vi "NET_1 (1).vi"() -> ()   [LabVIEW 2017]
uses:
  <vilib>/ErrorRing/Error Ring.xnode
panel:
  out "Gauge":dbl(knob) scale=0.0..10.0
  out "Array 2":dbl[](array[numeric])
  out "output array 2":dbl[][](array[numeric])
  out "Array":u32[](array[numeric])
  out "Numeric":u32
  out "subarray":string[](array[string])
  out "Trama":string[](array[string])
  in  "Al 3":bool
  in  "Al 2":bool
  in  "Al1":bool
  in  "Escribir":bool
  out "IsOpen":bool
  in  "stop":bool
  in  "Cerrar":bool
  in  "Abrir":bool
  in  "Puertos":string(combo)
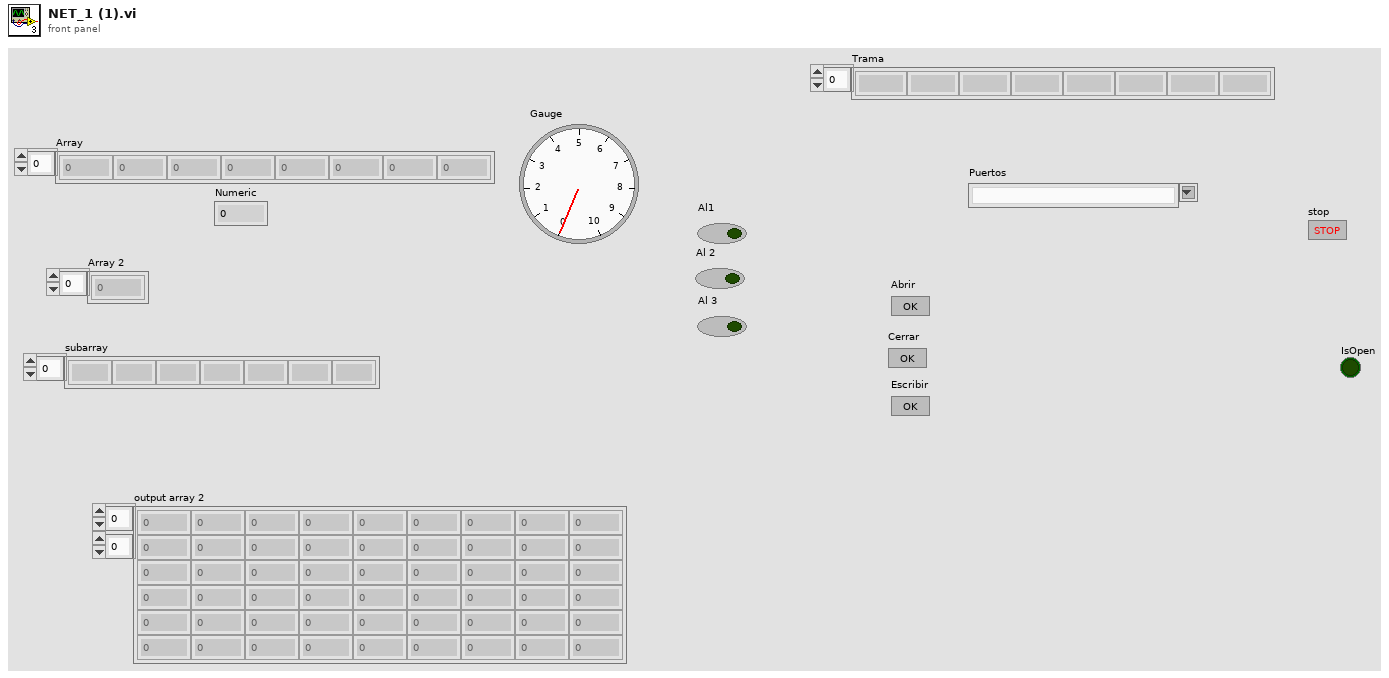
[diagram p1: front panel]
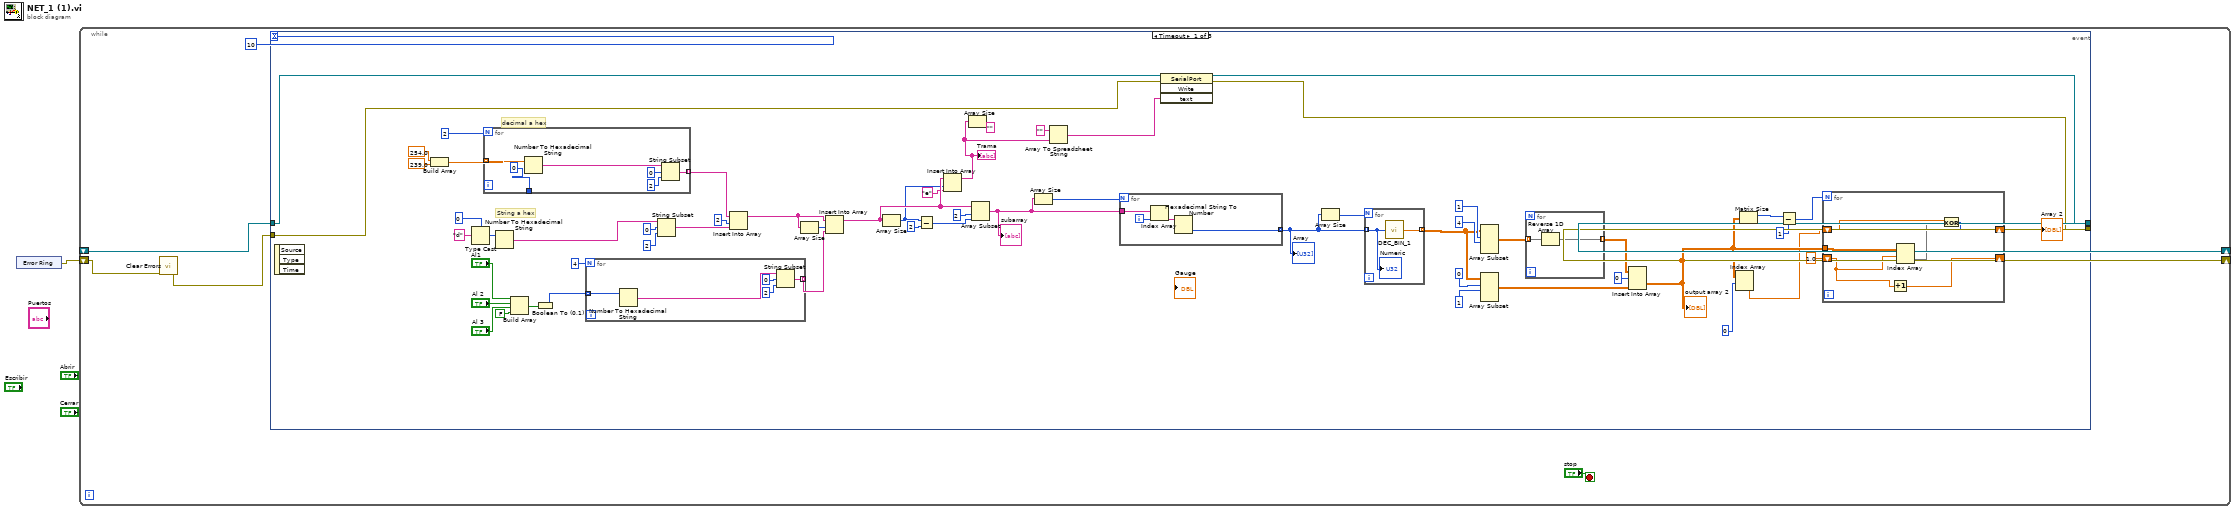
[diagram p0: block diagram]
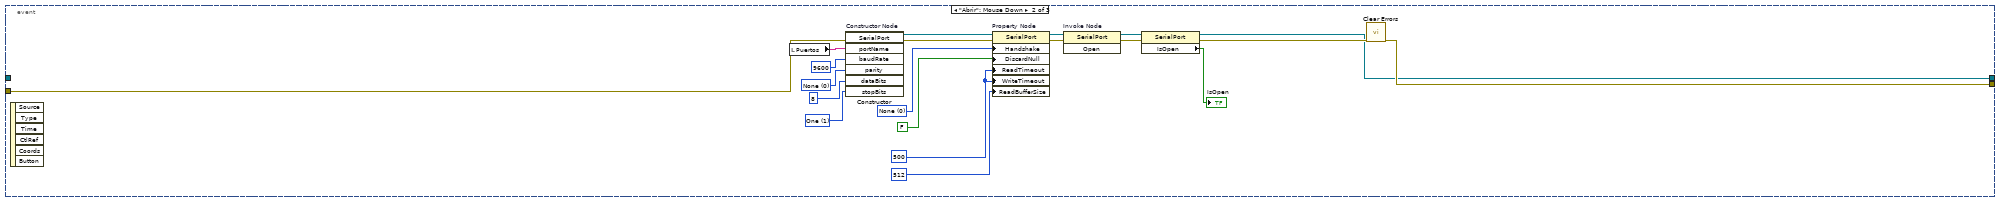
[diagram p2: hidden frame]
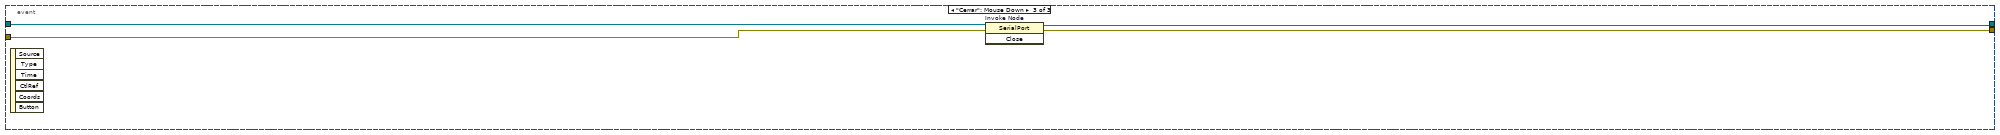
[diagram p3: hidden frame]
diagram:
  n1 = xnode "Error Ring"() -> ("error out"=w1:errorcluster)
  n2 = while {
    shift-right: [w7] -> _
    shift-left: _ -> [w5]
    shift-right: [w6] -> _
    shift-left: w1 -> [w4]
    stop <- "stop" stop-if-true
    n3 = call <vilib>:"Clear Errors.vi"("error in (no error)"=w4) -> ("error out"=w3:errorcluster)  [unwired: 5 in, 1 out]
    n4 = event shown="[0] Timeout" {
      selector: _ -> [_ _ _]
      dyn-events: _ -> [_ _ _]
      timeout: 10 -> [_ _ _]
      tunnel: [w11 w91 w111] -> w7
      tunnel: [w10 w93 w112] -> w6
      tunnel: w3 -> [w15 w94 w113]
      tunnel: w5 -> [w16 _ w114]
      event Timeout {
        (unwired) ""
        # "decimal a hex"
        # "String a hex"
        n5 = event-data() -> ()  [unwired: 1 in, 3 out]
        n6 = Build Array(254.0 ("element"), 239.0 ("element")) -> (w62:dbl[])
        n7 = Type Cast(type=0, x="d" ("String")) -> (*(type *) &x=w57:i32)
        n8 = for {
          N: 2 -> [_]
          tunnel: w62 -> [w87] mode=indexing
          tunnel: [w86] -> w55 mode=indexing
          tunnel: [0 ("offset")] -> _
          n9 = Number To Hexadecimal String(2:w87) -> (0:w90:string)  [unwired: 1 in]
          n10 = String Subset(string=w90, offset (0)=0, length (rest)=2 ("length (rest)")) -> (substring=w86:string)
        }
        n11 = Number To Hexadecimal String(2:w57) -> (0:w58:string)  [unwired: 1 in]
        n12 = Build Array("Al1", "Al 2", "Al 3", FALSE ("element")) -> (w48:bool[])
        n13 = Boolean To (0,1)(Boolean=w48) -> (0, 1=w47:i16[])
        n14 = for {
          N: 4 -> [_]
          tunnel: w47 -> [w82] mode=indexing
          tunnel: [w80] -> w46 mode=indexing
          n15 = Number To Hexadecimal String(2:w82) -> (0:w81:string)  [unwired: 1 in]
          n16 = String Subset(string=w81, offset (0)=0, length (rest)=2 ("length (rest)")) -> (substring=w80:string)
        }
        n17 = String Subset(string=w58, offset (0)=0, length (rest)=2 ("length (rest)")) -> (substring=w54:string)
        n18 = Insert Into Array "Insert Into Array"(array=w55, index=2, new element=w54) -> (w45:string[])
        n19 = Array Size(array=w45) -> (size(s)=w43:i32)
        n20 = Insert Into Array "Insert Into Array"(array=w45, index=w43, new element=w46) -> (w42:string[])
        n21 = Array Size(array=w42) -> (size(s)=w39:i32)
        n22 = Subtract(x=w39, y=2) -> (x-y=w37:i32)
        n23 = Insert Into Array "Insert Into Array"(array=w42, index=w39, new element="e" ("new element/subarray")) -> (w14:string[])
        "Trama" <- w14
        n24 = Array Size(array=w14) -> ()  [unwired: 1 out]
        n25 = Array Subset "Array Subset"(array=w42, index=2, length=w37) -> (w35:string[])
        "subarray" <- w35
        n26 = Array Size(array=w35) -> (size(s)=w36:i32)
        n27 = Array To Spreadsheet String(array=w14, 3:"" ("format string")) -> (spreadsheet string=w12:string)  [unwired: 1 in]
        n28 = for {
          N: w36 -> [_]
          tunnel: w35 -> [w79]
          tunnel: [w76] -> w33 mode=indexing
          i -> [w78]
          n29 = Index Array "Index Array"(array=w79, index=w78) -> (element=w77:string)
          n30 = Hexadecimal String To Number(string=w77) -> (number=w76:u32)  [unwired: 2 in, 1 out]
        }
        "Array" <- w33
        n31 = invoke class="SerialPort" method="Write"(reference=w16, error in=w15, "text"=w12) -> (reference out=w11:refnum<k24>, error out=w10:errorcluster)  [unwired: 1 in, 2 out]
        n32 = Array Size(array=w33) -> (size(s)=w34:i32)
        n33 = for {
          N: w34 -> [_]
          tunnel: w33 -> [w75] mode=indexing
          tunnel: [w74] -> w9 mode=indexing
          n34 = call "DEC_BIN_1.vi"("Numero Decimal"=w75) -> ("Binario"=w74:dbl[])
          "Numeric" <- w75
        }
        n35 = Array Subset "Array Subset"(array=w9, index (row)=1 ("index"), length (row)=4 ("length")) -> (w30:dbl[][])  [unwired: 2 in]
        n36 = Array Subset "Array Subset"(array=w9, index (row)=0 ("index"), length (row)=1 ("length")) -> (w25:dbl[][])  [unwired: 2 in]
        n37 = for {
          tunnel: w30 -> [w72] mode=indexing
          tunnel: [w73] -> w29 mode=indexing
          n38 = Reverse 1D Array(array=w72) -> (reversed array=w73:dbl[])
        }
        n39 = Insert Into Array "Insert Into Array"(array=w29, index (row)=0, new element=w25) -> (w22:dbl[][])  [unwired: 1 in]
        "output array 2" <- w22
        n40 = Index Array "Index Array"(array=w22, index (row)=0) -> (element=w18:dbl[])  [unwired: 1 in]
        n41 = Matrix Size(0:w22) -> (1:w21:i32)  [unwired: 1 out]
        n42 = Subtract(x=w21, y=1) -> (x-y=w19:i32)
        n43 = for {
          N: w19 -> [_]
          tunnel: w22 -> [w71]
          shift-right: [w69] -> w17
          shift-left: w18 -> [w68]
          shift-right: [w67] -> _
          shift-left: 1.0 -> [w66]
          n44 = Increment(x=w66) -> (x+1=w67:dbl)
          n45 = Index Array "Index Array"(array=w71, index (row)=w66) -> (element=w70:dbl[])  [unwired: 1 in]
          n46 = Exclusive Or(1:w70, 2:w68) -> (0:w69:i32[])
        }
        "Array 2" <- w17
      }
      event "Abrir": Mouse Down {
        w100 = 1 items=["None", "One", "Two", "OnePointFive"] ("stopBits")
        w102 = 0 items=["None", "Odd", "Even", "Mark", "Space"] ("parity")
        w105 = 500 ("ReadTimeout")
        w106 = 0 items=["None", "XOnXOff", "RequestToSend", "RequestToSendXOnXOff"] ("Handshake")
        n47 = event-data() -> ()  [unwired: 1 in, 6 out]
        n48 = local read "Puertos"() -> (w99:string)
        n49 = constructor on="Constructor Node" class="SerialPort"(error in=w94, "portName"=w99, "baudRate"=9600, "parity"=w102, "dataBits"=8, "stopBits"=w100) -> (reference out=w110:refnum<k24>, error out=w108:errorcluster)  [unwired: 2 in, 6 out]
        n50 = property on="Property Node" class="SerialPort"(reference=w110, error in=w108, "Handshake"=w106, "DiscardNull"=FALSE, "ReadTimeout"=w105, "WriteTimeout"=w105, "ReadBufferSize"=512 ("ReadTimeout")) -> (reference out=w109:refnum<k24>, error out=w107:errorcluster)
        n51 = invoke on="Invoke Node" class="SerialPort" method="Open"(reference=w109, error in=w107) -> (reference out=w97:refnum<k24>, error out=w96:errorcluster)  [unwired: 1 in, 1 out]
        n52 = property class="SerialPort"(reference=w97, error in=w96) -> (reference out=w91:refnum<k24>, error out=w92:errorcluster, "IsOpen"=→"IsOpen":bool)
        n53 = call <vilib>:"Clear Errors.vi"("error in (no error)"=w92) -> ("error out"=w93:errorcluster)  [unwired: 5 in, 1 out]
      }
      event "Cerrar": Mouse Down {
        n54 = event-data() -> ()  [unwired: 1 in, 6 out]
        n55 = invoke on="Invoke Node" class="SerialPort" method="Close"(reference=w114, error in=w113) -> (reference out=w111:refnum<k24>, error out=w112:errorcluster)  [unwired: 1 in, 1 out]
      }
    }
  }
